vi "DSF.Shared.Configuration.Framework.Initialize.vi"(6 "Cycle Timing Factors":T1={"Decimation"=1, "Offset"=0}, 7 "Custom Parameters":variant, 8 "error in (no error)":errorcluster, 9 "Plugin Configurations":refnum<class "DSF.Shared.Configuration.Plugin.lvclass">[](array[class]), 10 "Name":string, 11 "Framework Configuration in":refnum<class "DSF.Shared.Configuration.Framework.lvclass">) -> (0 "error out":errorcluster, 3 "Framework Configuration out":refnum<class "DSF.Shared.Configuration.Framework.lvclass">)   [LabVIEW 2016, in "DSF.Shared.lvlib" / "DSF.Shared.Configuration.Framework.lvclass"]
uses:
  DSF.Shared.Configuration.Framework.lvclass
  C:/Git/SourceTree/DSF/Source/Shared/Classes/Configuration/DSF.Shared.Configuration.Cycle Timed.lvclass
  Plugin/DSF.Shared.Configuration.Plugin.lvclass
  Typedefs/DSF.Shared.Typedefs.Cycle Timing Factors.ctl
  DSF.Shared.Configuration.Framework.lvclass/DSF.Shared.Configuration.Framework.ctl
  Configuration/DSF.Shared.Configuration.Cycle Timed.lvclass
  DSF.Shared.lvlib
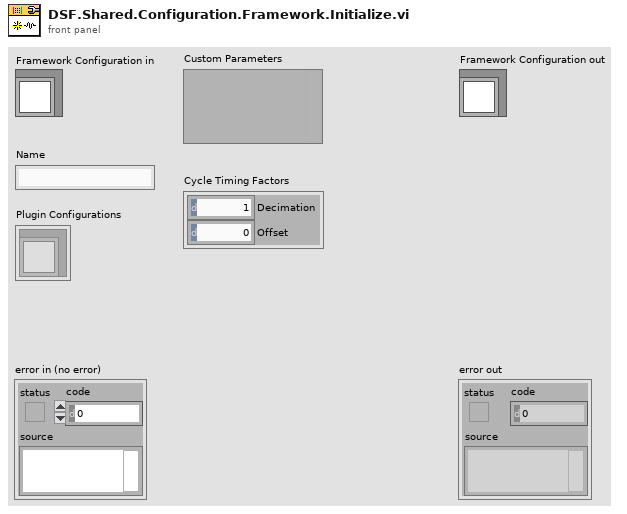
[diagram p1: front panel]
types:
  T1 = typedef "DSF.Shared.lvlib/DSF.Shared.Typedefs.Cycle Timing Factors.ctl" = cluster{"Decimation":u64, "Offset":u64}
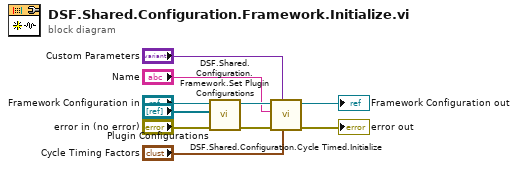
[diagram p0: block diagram]
diagram:
  n1 = call "DSF.Shared.Configuration.Framework.Set Plugin Configurations.vi"("error in (no error)"="error in (no error)", "Plugin Configurations"="Plugin Configurations", "Framework Configuration in"="Framework Configuration in") -> ("error out"=w7:errorcluster, "Framework Configuration out"=w6:refnum<class "DSF.Shared.Configuration.Framework.lvclass">)  [unwired: 7 in]
  n2 = call "DSF.Shared.Configuration.Cycle Timed.Initialize.vi"("Cycle Timing Factors"="Cycle Timing Factors", "Custom Parameters"="Custom Parameters", "error in (no error)"=w7, "Name"="Name", "Cycle Timed Configuration in"=w6) -> ("error out"=→"error out":errorcluster, "Cycle Timed Configuration out"=→"Framework Configuration out":refnum<class "DSF.Shared.Configuration.Framework.lvclass">)  [unwired: 5 in]
